vi "AR-DO-create.vi"(8 "error in":errorcluster, 11 "lines":tag="Dev1/port0/line0:3") -> (0 "error out":errorcluster, 3 "DO task out":refnum<k21>)   [LabVIEW 2021]
uses:
  <vilib>/DAQmx/create/channels.llb/DAQmx Create Channel (DO-Digital Output).vi
  <resource>/objmgr/daqmx.rc
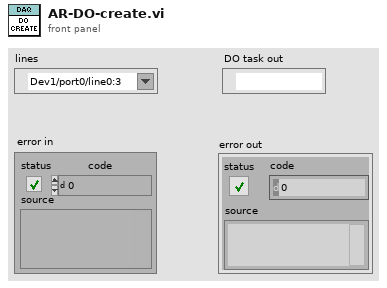
[diagram p1: front panel]
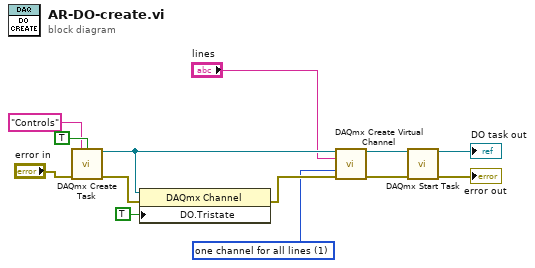
[diagram p0: block diagram]
diagram:
  w5 = 1 items=["one channel for each line", "one channel for all lines"] ("line grouping")
  n1 = call <vilib>:"DAQmx Create Task.vi"("new task name"="Controls", "auto cleanup"=TRUE, "error in"="error in") -> ("task out"=w9:refnum<k21>, "error out"=w8:errorcluster)  [unwired: 11 in]
  n2 = property class="DAQmx Channel"(reference=w9, error in=w8, "DO.Tristate"=TRUE) -> (error out=w10:errorcluster)  [unwired: 1 out]
  n3 = call-poly <vilib>:"DAQmx Create Virtual Channel.vi"("task in"=w9, "lines"="lines", "line grouping"=w5, "error in"=w10) -> ("task out"=w6:refnum<k21>, "error out"=w11:errorcluster)  [unwired: 10 in]
  n4 = call <vilib>:"DAQmx Start Task.vi"("task/channels in"=w6, "error in"=w11) -> ("task out"=→"DO task out":refnum<k21>, "error out"=→"error out":errorcluster)  [unwired: 12 in]
